vi "Scale Reading Percision.vi"(0 "VISA resource name":refnum<visa-resource-name>) -> (4 "read buffer":string)   [LabVIEW 2009]
uses:
  <vilib>/Instr/_visa.llb/VISA Configure Serial Port (Instr).vi
panel:
  out "Stable":bool
  out "error out":errorcluster
  in  "Zero":bool=TRUE
  in  "stop":bool
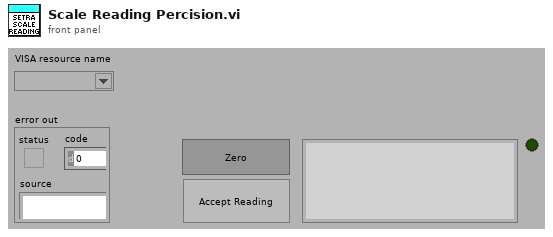
[diagram p1: front panel]
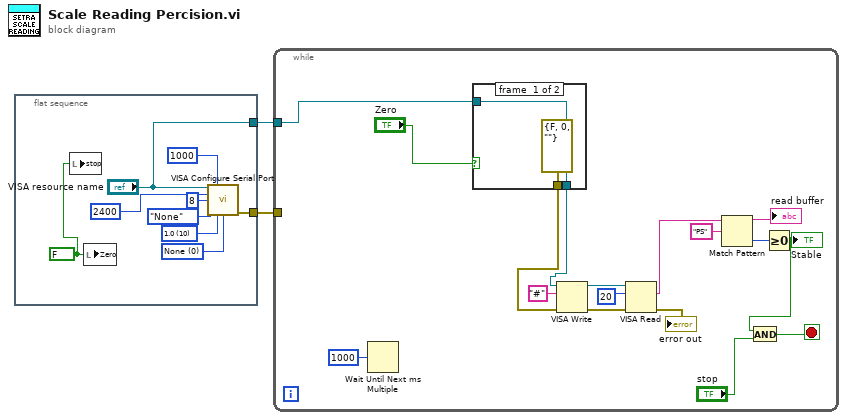
[diagram p0: block diagram]
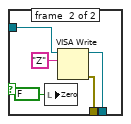
[diagram p2: hidden frame]
diagram:
  n1 = flat-sequence {
    tunnel: [w5] -> w2
    tunnel: ["VISA resource name"] -> w1
    frame #0 {
      w3 = FALSE ("Zero")
      w7 = u16 0 items=["None", "XON/XOFF", "RTS/CTS", "XON/XOFF & RTS/CTS", "DTR/DSR", "XON/XOFF & DTR/DSR"] ("flow control (0:none)")
      w8 = u16 10 items=["1.0"=10, "1.5"=15, "2.0"=20] ("stop bits (10: 1 bit)")
      n2 = local write "stop"(w3) -> ()
      n3 = local write "Zero"(w3) -> ()
      n4 = call-poly "VISA Configure Serial Port"("VISA resource name"="VISA resource name", "timeout (10sec)"=u32 1000, "baud rate (9600)"=u32 2400, "data bits (8)"=u16 8, "parity (0:none)"=enum16{"None", "Odd", "Even", "Mark", "Space"}."None", "stop bits (10: 1 bit)"=w8, "flow control (0:none)"=w7) -> ("error out"=w5:errorcluster)  [unwired: 7 in, 1 out]
    }
  }
  n5 = while {
    tunnel: w2 -> [_]
    tunnel: w1 -> [w27]
    stop <- w13 stop-if-true
    n6 = Wait Until Next ms Multiple(millisecond multiple=u32 1000) -> ()  [unwired: 1 out]
    n7 = case shown="True" "Zero" {
      tunnel: w27 -> [w30 w35]
      tunnel: [w30 w33] -> w21
      tunnel: [errorcluster {"status"=FALSE, "code"=0, "source"=""} ("error out") w32] -> w20
      frame #0 {
      }
      frame #1 {
        n8 = local write "Zero"(FALSE ("Zero")) -> ()
        n9 = VISA Write(VISA resource name=w35, write buffer="Z") -> (VISA resource name out=w33:refnum<visa-resource-name>, error out=w32:errorcluster)  [unwired: 1 in, 1 out]
      }
    }
    n10 = VISA Write(VISA resource name=w21, write buffer="#", error in (no error)=w20) -> (VISA resource name out=w23:refnum<visa-resource-name>, error out=w22:errorcluster)  [unwired: 1 out]
    n11 = VISA Read(VISA resource name=w23, byte count=u32 20, error in (no error)=w22) -> (read buffer=w18:string, error out=→"error out":errorcluster)  [unwired: 2 out]
    n12 = Match Pattern(string=w18, regular expression="PS") -> (before substring=→"read buffer":string, offset past match=w15:i32)  [unwired: 1 in, 2 out]
    n13 = Greater Or Equal To 0?(x=w15) -> (x >= 0?=w12:bool)
    "Stable" <- w12
    n14 = And(x=w12, y="stop") -> (x .and. y?=w13:bool)
  }
